vi "Write State.vi"(8 "error in (no error)":errorcluster, 10 "OpMode-NP":T1, 11 "Container in":refnum<class "Container.lvclass">) -> (0 "error out":errorcluster, 3 "Container out":refnum<class "Container.lvclass">)   [LabVIEW 2016, in "Container.lvclass"]
uses:
  Container.lvclass
  Controls/Operational Modes.ctl
  Controls/Shutter States.ctl
  Container.lvclass/Container.ctl
  ExtFlat/ExtFlatShutt.lvclass
  LFCSim/LFCSimShutt.lvclass
  Sci/SciShutt.lvclass
  SimFlat/SimFlatShutt.lvclass
  Solar/SolarShutt.lvclass
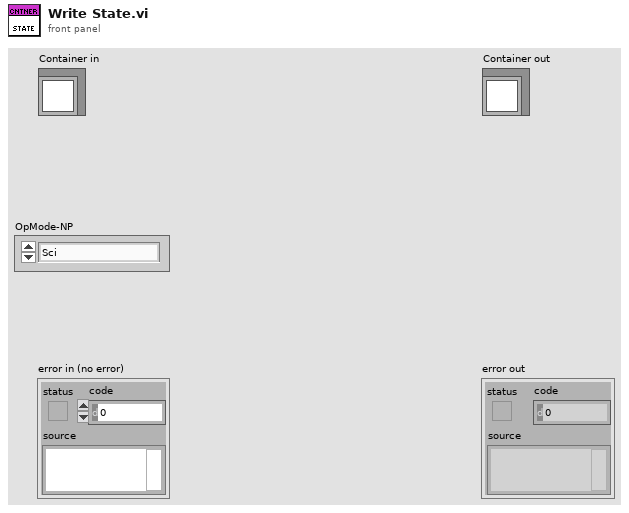
[diagram p1: front panel]
types:
  T1 = typedef "Operational Modes.ctl" = enum16{"Sci", "Sci-LFC", "Solar", "Solar-LFC", "LFC", "LFC-Sim", "LFC-Both", "ThAr", "ThAr-LFC", "Flat", "ExtFlat", "ExtFlat-Sim", "ExtFlat-Both", "Qtz", "ExtQtz", "ExtQtz-Sim", "ExtQtz-Both", "Dark", "Manual", "Off"}
  T2 = typedef "Shutter States.ctl" = enum16{"Open", "Close", "Wait", "Off", "Arm", "Idle"}
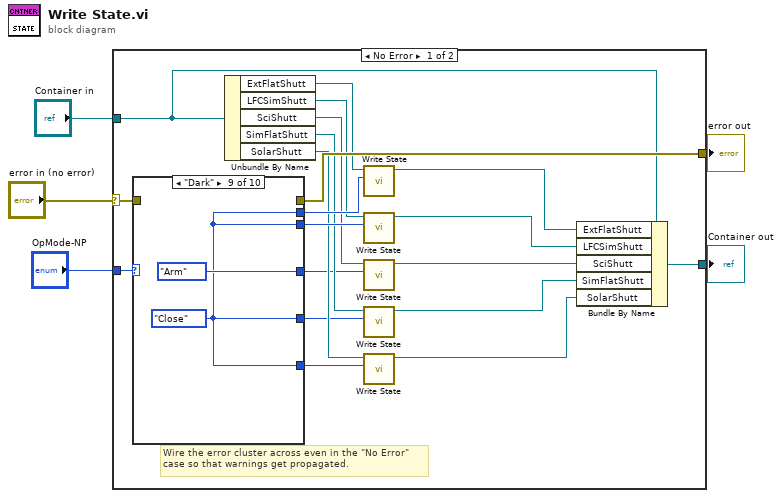
[diagram p0: block diagram]
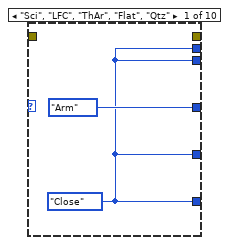
[diagram p2: hidden frame]
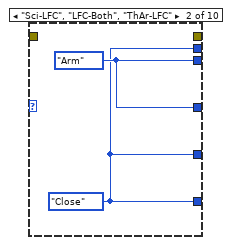
[diagram p3: hidden frame]
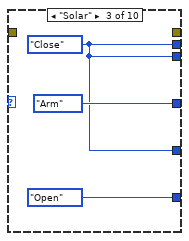
[diagram p4: hidden frame]
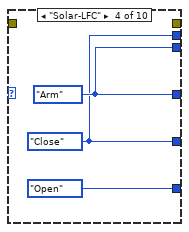
[diagram p5: hidden frame]
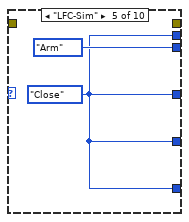
[diagram p6: hidden frame]
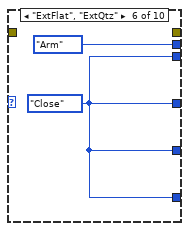
[diagram p7: hidden frame]
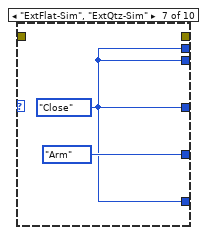
[diagram p8: hidden frame]
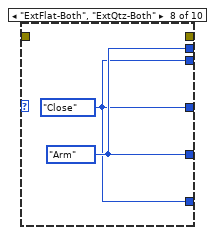
[diagram p9: hidden frame]
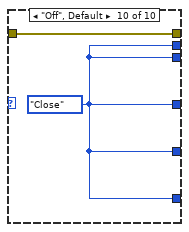
[diagram p10: hidden frame]
diagram:
  n1 = case shown="No Error" "error in (no error)" {
    selector: "error in (no error)" -> [w24 w49]
    tunnel: [w23 w49] -> w4
    tunnel: [w14 w48] -> w2
    tunnel: "Container in" -> [w13 w48]
    tunnel: "OpMode-NP" -> [w25 _]
    frame No Error {
      # "Wire the error cluster across even in the \"No Error\"\ncase so that warnings get propagated."
      n2 = case shown="\"Dark\"" w25 {
        tunnel: [Shutter_States."Arm" ("Set") w29 Shutter_States."Arm" ("Set") w35 w36 w38 w40 w42 Shutter_States."Arm" ("Set") w47] -> w7
        tunnel: [w26 w29 w31 w35 Shutter_States."Arm" ("Set") w38 w40 w42 w44 w47] -> w19
        tunnel: [w26 w28 w31 w34 w36 Shutter_States."Arm" ("Set") w40 w43 w44 w47] -> w21
        tunnel: [w26 w28 w31 w34 w36 w38 Shutter_States."Arm" ("Set") w43 w44 w47] -> w15
        tunnel: [w26 w28 Shutter_States."Open" ("Set") Shutter_States."Open" ("Set") w36 w38 w40 w42 w44 w47] -> w16
        tunnel: w24 -> [_ _ _ _ _ _ _ _ _ w46]
        tunnel: [_ _ _ _ _ _ _ _ _ w46] -> w23
        frame "Sci", "LFC", "ThAr", "Flat", "Qtz" {
          w26 = Shutter_States."Close" ("Set")
        }
        frame "Sci-LFC", "LFC-Both", "ThAr-LFC" {
          w28 = Shutter_States."Close" ("Set")
          w29 = Shutter_States."Arm" ("Set")
        }
        frame "Solar" {
          w31 = Shutter_States."Close" ("Set")
        }
        frame "Solar-LFC" {
          w34 = Shutter_States."Close" ("Set")
          w35 = Shutter_States."Arm" ("Set")
        }
        frame "LFC-Sim" {
          w36 = Shutter_States."Close" ("Set")
        }
        frame "ExtFlat", "ExtQtz" {
          w38 = Shutter_States."Close" ("Set")
        }
        frame "ExtFlat-Sim", "ExtQtz-Sim" {
          w40 = Shutter_States."Close" ("Set")
        }
        frame "ExtFlat-Both", "ExtQtz-Both" {
          w42 = Shutter_States."Close" ("Set")
          w43 = Shutter_States."Arm" ("Set")
        }
        frame "Dark" {
          w44 = Shutter_States."Close" ("Set")
        }
        frame "Off", Default {
          w47 = Shutter_States."Close" ("Set")
        }
      }
      n3 = Unbundle By Name(w13) -> ("ExtFlatShutt"=w22:refnum<class "ExtFlatShutt.lvclass">, "LFCSimShutt"=w20:refnum<class "LFCSimShutt.lvclass">, "SciShutt"=w8:refnum<class "SciShutt.lvclass">, "SimFlatShutt"=w18:refnum<class "SimFlatShutt.lvclass">, "SolarShutt"=w17:refnum<class "SolarShutt.lvclass">)
      n4 = call-dynamic "Write State.vi"("Set"=w21, "Shutter in"=w22) -> ("Shutter out"=w9:refnum<class "ExtFlatShutt.lvclass">)  [unwired: 8 in, 1 out]
      n5 = call-dynamic "Write State.vi"("Set"=w19, "Shutter in"=w20) -> ("Shutter out"=w10:refnum<class "LFCSimShutt.lvclass">)  [unwired: 8 in, 1 out]
      n6 = call-dynamic "Write State.vi"("Set"=w7, "Shutter in"=w8) -> ("Shutter out"=w6:refnum<class "SciShutt.lvclass">)  [unwired: 8 in, 1 out]
      n7 = call-dynamic "Write State.vi"("Set"=w15, "Shutter in"=w18) -> ("Shutter out"=w11:refnum<class "SimFlatShutt.lvclass">)  [unwired: 8 in, 1 out]
      n8 = call-dynamic "Write State.vi"("Set"=w16, "Shutter in"=w17) -> ("Shutter out"=w12:refnum<class "SolarShutt.lvclass">)  [unwired: 8 in, 1 out]
      n9 = Bundle By Name(cluster=w13, "ExtFlatShutt"=w9, "LFCSimShutt"=w10, "SciShutt"=w6, "SimFlatShutt"=w11, "SolarShutt"=w12) -> (w14:refnum<class "Container.lvclass">)
    }
    frame Error {
    }
  }
  "error out" <- w4
  "Container out" <- w2
